vi "RTread.vi"(0 "FPGA VI Reference In":refnum<k20>, 1 "error in":errorcluster) -> (2 "Blk Pos (in)":sgl, 3 "Blk Pos (Amp)":sgl, 4 "Torque Pin (Amp)":sgl, 6 "Load 1 (lbf)":sgl, 7 "RPM 1":dbl, 8 "Load 2 (lbf)":sgl, 9 "RPM 2":dbl, 10 "Load 1 (V)":sgl, 11 "Tach 1 Period (ms)":sgl, 12 "Load 2 (V)":sgl, 13 "Tach 2 Period (ms)":sgl, 14 "FPGA VI Reference Out":refnum<k20>, 15 "error out":errorcluster, 16 "Blk Pos (ft)":dbl, 17 "Total Load (lbf)":sgl, 18 "Torque (ft-lbf)":sgl, 19 "RPM":dbl)   [LabVIEW 2019]
uses:
  <vilib>/Utility/error.llb/Error Cluster From Error Code.vi
  <vilib>/rvi/errors/niLvFpgaAdjustHostInterfaceError.vi
  <vilib>/rvi/interface/nirviMethod/nirviMethod.xnode
  <vilib>/FPGAPlugInAG/Dynamic/niLvFpga_ReadFifo_Dynamic.vi
  <vilib>/rvi/errors/niLvFpgaMergeErrorWithErrorCode.vi
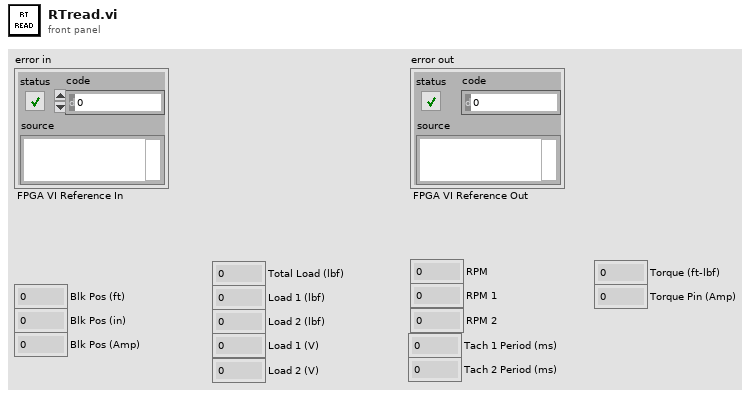
[diagram p1: front panel]
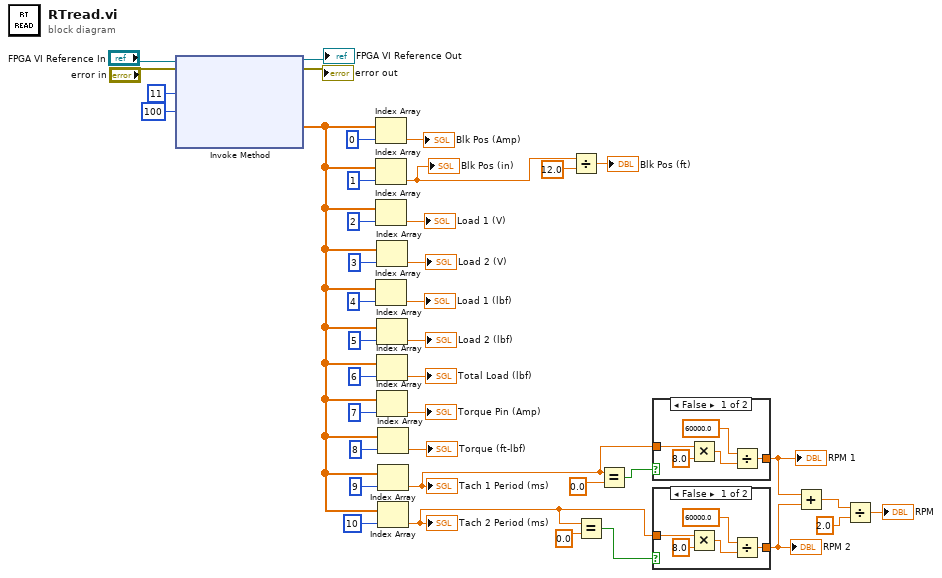
[diagram p0: block diagram]
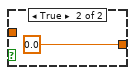
[diagram p2: hidden frame]
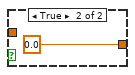
[diagram p3: hidden frame]
diagram:
  n1 = xnode "Invoke Method"("FPGA VI Reference In"="FPGA VI Reference In", "error in"="error in", "Number of Elements"=u32 11, "Timeout (ms)"=100) -> ("FPGA VI Reference Out"=→"FPGA VI Reference Out":refnum<k20>, "error out"=→"error out":errorcluster, "Data"=w21:sgl[])  [unwired: 1 out]
  n2 = Index Array(array=w21, index=0) -> (element=→"Blk Pos (Amp)":sgl)
  n3 = Index Array(array=w21, index=1) -> (element=w17:sgl)
  "Blk Pos (in)" <- w17
  n4 = Index Array(array=w21, index=2) -> (element=→"Load 1 (V)":sgl)
  n5 = Index Array(array=w21, index=4) -> (element=→"Load 1 (lbf)":sgl)
  n6 = Index Array(array=w21, index=3) -> (element=→"Load 2 (V)":sgl)
  n7 = Index Array(array=w21, index=5) -> (element=→"Load 2 (lbf)":sgl)
  n8 = Index Array(array=w21, index=6) -> (element=→"Total Load (lbf)":sgl)
  n9 = Index Array(array=w21, index=7) -> (element=→"Torque Pin (Amp)":sgl)
  n10 = Index Array(array=w21, index=8) -> (element=→"Torque (ft-lbf)":sgl)
  n11 = Index Array(array=w21, index=9) -> (element=w4:sgl)
  "Tach 1 Period (ms)" <- w4
  n12 = Index Array(array=w21, index=10) -> (element=w1:sgl)
  "Tach 2 Period (ms)" <- w1
  n13 = Divide(x=w17, y=sgl 12.0) -> (x/y=→"Blk Pos (ft)":sgl)
  n14 = Equal?(x=w1, y=0.0) -> (x = y?=w2:bool)
  n15 = Equal?(x=w4, y=0.0) -> (x = y?=w3:bool)
  n16 = case shown="False" w3 {
    tunnel: w4 -> [w44 _]
    tunnel: [w41 sgl 0.0] -> w7
    frame False {
      n17 = Multiply(x=w44, y=sgl 8.0) -> (x*y=w43:sgl)
      n18 = Divide(x=sgl 60000.0 ("y"), y=w43) -> (x/y=w41:sgl)
    }
    frame True {
    }
  }
  "RPM 1" <- w7
  n19 = case shown="False" w2 {
    tunnel: w1 -> [w50 _]
    tunnel: [w47 sgl 0.0] -> w6
    frame False {
      n20 = Multiply(x=w50, y=sgl 8.0) -> (x*y=w49:sgl)
      n21 = Divide(x=sgl 60000.0 ("y"), y=w49) -> (x/y=w47:sgl)
    }
    frame True {
    }
  }
  "RPM 2" <- w6
  n22 = Add(x=w7, y=w6) -> (x+y=w9:sgl)
  n23 = Divide(x=w9, y=sgl 2.0) -> (x/y=→"RPM":sgl)
